vi "3dgraph.vi"() -> ()   [LabVIEW 2020]
uses:
  <vilib>/picture/3D Picture Control/Object/Create Object (drawable).vi
  <vilib>/picture/3D Picture Control/NI_3D Picture Control.lvlib
panel:
  out "3D Picture":refnum<vi>(3d-picture)
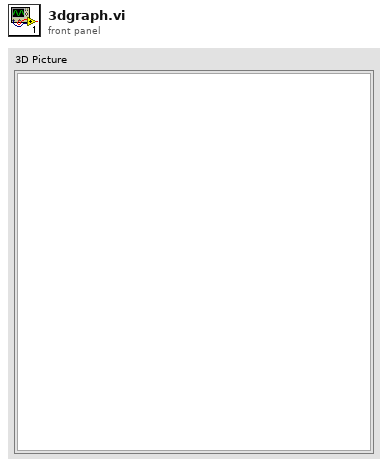
[diagram p1: front panel]
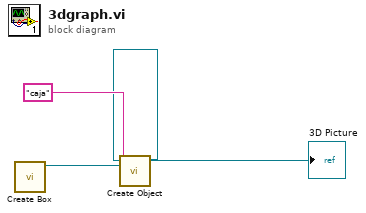
[diagram p0: block diagram]
diagram:
  n1 = call <vilib>:"Create Box.vi"() -> ("New Box Refnum"=w3:refnum<vi>)  [unwired: 10 in, 1 out]
  n2 = call-poly <vilib>:"Create Object.vi"("Geometry"=w3, "Name"="caja") -> ("Scene:New Object"=→"3D Picture":refnum<vi>)  [unwired: 8 in, 1 out]
